vi "Bc&gfactor.vi"(4 "R square":cluster{dbl, dbl}[](graph)=[{-90000.0, 0.9936483367603044}, {-87906.97674418605, 0.9950094850030079}, {-85813.95348837209, 0.9957274737690295}, {-83720.93023255814, 0.9933108814011996}, {-81627.90697674418, 0.992357867872986}, {-79534.88372093023, 0.9862292416058566}, {-77441.86046511628, 0.99627541563675}, {-75348.83720930232, 0.9780001446047889}, {-73255.81395348837, 0.9762525196246166}, {-71162.79069767441, 0.9805623164953412}, {-69069.76744186046, 0.9733364259427615}, {-66976.7441860465, 0.9866906891307189}, {-64883.72093023256, 0.9887677477278096}, {-62790.6976744186, 0.9647771076841904}, {-60697.67441860465, 0.9547794787863182}, {-58604.651162790695, 0.9942809429807753}, {-56511.62790697674, 0.9851661179243407}, {-54418.60465116279, 0.9686064936549159}, {-52325.58139534883, 0.9659153710307546}, {-50232.55813953488, 0.9617268214492714}, {-48139.534883720924, 0.9756720636568874}, {-46046.51162790697, 0.9839504663053658}, {-43953.488372093016, 0.9970014960760687}, {-41860.46511627906, 0.9884092692332003}, {-39767.441860465115, 0.9866795475083417}, {-37674.41860465116, 0.9905062595043629}, {-35581.395348837206, 0.9798470326477143}, {-33488.37209302325, 0.9763040209572704}, {-31395.348837209298, 0.9974412233607519}, {-29302.325581395344, 0.9790950602168367}, {-27209.30232558139, 0.985787657243487}, {-25116.279069767435, 0.994663632255808}, {-23023.25581395348, 0.9948455965833045}, {-20930.232558139527, 0.9957582677028887}, {-18837.209302325573, 0.9958266077752963}, {-16744.18604651162, 0.9907170020986631}, {-14651.162790697665, 0.9943927190181459}, {-12558.13953488371, 0.9926116840879449}, {-10465.116279069756, 0.9936118308328861}, {-8372.093023255802, 0.993852544818158}, {-6279.069767441848, 0.991095330580116}, {-4186.046511627894, 0.9915888136201866}, {-2093.0232558139396, 0.9952686470079972}, {1.4551915228366852e-11, 0.9951187760658085}, {2093.0232558139687, 0.9938327422163827}, {4186.046511627923, 0.9949656993934944}, {6279.069767441877, 0.9912005637296157}, {8372.093023255831, 0.9916696176817267}, {10465.11627906977, 0.9922195047323839}, {12558.139534883725, 0.9929868887027957}, {14651.16279069768, 0.9900196190607464}, {16744.186046511633, 0.9944283927116259}, {18837.209302325587, 0.9940419981816503}, {20930.23255813954, 0.9927548489146202}, {23023.255813953496, 0.9936445754738522}, {25116.27906976745, 0.9980677514433665}, {27209.302325581404, 0.9960253172243516}, {29302.32558139536, 0.9927559692084316}, {31395.348837209312, 0.9773515443784792}, {33488.37209302327, 0.9897212577220764}, {35581.39534883722, 0.9924602641830366}, {37674.418604651175, 0.9791788400015979}, {39767.44186046513, 0.9788017425910343}, {41860.46511627908, 0.9808865900675626}, {43953.48837209304, 0.9789571284233267}, {46046.51162790699, 0.9671045339132186}, {48139.534883720946, 0.9672112912864314}, {50232.5581395349, 0.9665854302890936}, {52325.581395348854, 0.9620995151108727}, {54418.60465116281, 0.9860375825085537}, {56511.62790697676, 0.9877298129618225}, {58604.65116279072, 0.9625519591858813}, {60697.67441860467, 0.9721292461291907}, {62790.697674418625, 0.9759515933730254}, {64883.72093023258, 0.9762546173916274}, {66976.74418604653, 0.9914257931857835}, {69069.76744186049, 0.9589212650542382}, {71162.79069767444, 0.7584191634223125}, {73255.8139534884, 0.975789027366707}, {75348.83720930235, 0.9825220775303888}, {77441.8604651163, 0.9890951437370847}, {79534.88372093026, 0.9695146827415762}, {81627.90697674421, 0.9879709487631367}, {83720.93023255817, 0.9877215091218606}, {85813.95348837212, 0.9938806771671042}, {87906.97674418607, 0.9847409146593209}], 8 "Coupling factor error":dbl, 9 "Coupling factor (eV/V)":dbl=0.1, 10 "Which splitting?":i32, 11 "XY Graph 4":cluster{dbl[], dbl[]}[](graph)=[{[-0.02736853412017211, -0.02736853412017211, -0.027457159682098792, -0.02714680119515219, -0.027446691867251106, -0.02737107022650992, -0.027461949140044236, -0.027256401341539064, -0.026844150670273844, -0.027419393193521695, -0.027303914098034662, -0.02703602857347208, -0.026888259949045673, -0.026790317754302132, -0.026790317754302132, -0.026707850548493665, -0.026570137455754914, -0.026515227867687362, -0.026658413988083815, -0.02635338740252281, -0.026267451338723564, -0.026280953558885083, -0.026109172200008007, -0.025812412430651806, -0.02584267749186701, -0.02582141266526132, -0.025807417699267175, -0.025801332345852277, -0.025821043911205325, -0.025805086007194167, -0.025791278388417656, -0.025772190934840334, -0.02548288242077668, -0.025336678648638575, -0.02567859725920492, -0.0251601862977569, -0.025085545468475877, -0.025013386768161117, -0.024935335121923342, -0.02736853412017211, -0.027457159682098792, -0.027574435649012727, -0.027554636167478386, -0.027551280185925644, -0.02791992364189102, -0.027503183763744384, -0.027618288300652723, -0.027446691867251106, -0.0277547695215205, -0.02760603475092372, -0.027461949140044236, -0.027522335544211626, -0.027503918369851946, -0.027419393193521695, -0.027303914098034662, -0.028033474343692046, -0.02804592066528165, -0.028006221411939727, -0.028006221411939727, -0.028207245954529003, -0.028279854967391334, -0.028432698354546673, -0.028674911642963354, -0.028695367509489752, -0.028788991538842516, -0.028859733108892546, -0.028885909800132156, -0.02931385357599471, -0.02883940989296912, -0.029107906174069182, -0.02914731021476181, -0.02920151841150575, -0.02863587278290227, -0.0295034906955593, -0.02997153941497236, -0.029743359934365898, -0.029820070650600022, -0.02951890711445811, -0.029555073471882756, -0.03004045441204873, -0.030156155658522733, -0.03027418428153998, -0.03011762696127086, -0.02736853412017211, -0.02757948642923058, -0.027610051126103378, -0.02764371579608451, -0.02756195552606243, -0.027634391513683045, -0.0275993752474062, -0.027127858278431297, -0.027440893163395392, -0.02744279598938577, -0.0275929298338454, -0.027591913990705083, -0.027565176585148243, -0.027533400296601417, -0.027330808874349643, -0.026744397861130295, -0.026982223848265225, -0.0269200804791046, -0.026856856233696994, -0.026700905436478503, -0.026700905436478503, -0.026665888611385614, -0.026544473254661284, -0.026445905848945565, -0.026338442772813758, -0.026263987266378474, -0.026551732521948368, -0.025944373776851146, -0.026112993018050888, -0.025889198816972006, -0.02586884204773503, -0.02588741873327973, -0.02585416095870263, -0.025896027615352635, -0.02588651620829451, -0.025899204618664493, -0.02586615626570455, -0.025770624667800432, -0.025703440860855863, -0.025747957866592296, -0.02535208231276207, -0.0252641528372817, -0.02521204130779185, -0.025156133749437332, -0.028319357512760632, -0.028373870368935062, -0.02800141524302324, -0.02756195552606243, -0.027634391513683045, -0.0275993752474062, -0.027689782895953863, -0.027826807607735864, -0.027950048307487676, -0.0275929298338454, -0.027591913990705083, -0.027565176585148243, -0.027533400296601417, -0.028298889889664804, -0.028307392754636704, -0.0283834573520277, -0.028475963804310153, -0.028508912222203024, -0.028508912222203024, -0.028646314658785015, -0.028200351086857745, -0.0287555540748013, -0.02873971887513881, -0.028779787878370027, -0.029072053575197022, -0.02895116220904841, -0.029287108790671378, -0.029178204968174144, -0.029322294689052453, -0.029417108027244444, -0.029433069816662265, -0.02962878437629653, -0.029718349543882774, -0.029788089545410783, -0.02987921181622441, -0.029600956616660113, -0.02905050167349195, -0.02917031235640807, -0.03011604320884724, -0.030126554480480978, -0.030182798802889002, -0.030209271213091124], [0.0, 1.4551915228366852e-11, 2093.0232558139687, 14651.16279069768, 16744.186046511633, 18837.209302325587, 23023.255813953496, 25116.27906976745, 27209.302325581404, 29302.32558139536, 31395.348837209312, 33488.37209302327, 35581.39534883722, 37674.418604651175, 37674.418604651175, 39767.44186046513, 41860.46511627908, 43953.48837209304, 46046.51162790699, 48139.534883720946, 50232.5581395349, 52325.581395348854, 54418.60465116281, 56511.62790697676, 58604.65116279072, 60697.67441860467, 62790.697674418625, 64883.72093023258, 66976.74418604653, 69069.76744186049, 71162.79069767444, 73255.8139534884, 75348.83720930235, 77441.8604651163, 79534.88372093026, 81627.90697674421, 83720.93023255817, 85813.95348837212, 87906.97674418607, 1.4551915228366852e-11, 2093.0232558139687, 4186.046511627923, 6279.069767441877, 8372.093023255831, 10465.11627906977, 12558.139534883725, 14651.16279069768, 16744.186046511633, 18837.209302325587, 20930.23255813954, 23023.255813953496, 25116.27906976745, 27209.302325581404, 29302.32558139536, 31395.348837209312, 33488.37209302327, 35581.39534883722, 37674.418604651175, 37674.418604651175, 39767.44186046513, 41860.46511627908, 43953.48837209304, 46046.51162790699, 48139.534883720946, 50232.5581395349, 52325.581395348854, 54418.60465116281, 56511.62790697676, 58604.65116279072, 60697.67441860467, 62790.697674418625, 64883.72093023258, 66976.74418604653, 69069.76744186049, 71162.79069767444, 73255.8139534884, 75348.83720930235, 77441.8604651163, 79534.88372093026, 81627.90697674421, 83720.93023255817, 85813.95348837212, 87906.97674418607, 0.0, -2093.0232558139396, -4186.046511627894, -6279.069767441848, -10465.116279069756, -12558.13953488371, -14651.162790697665, -16744.18604651162, -18837.209302325573, -20930.232558139527, -23023.25581395348, -25116.279069767435, -27209.30232558139, -29302.325581395344, -31395.348837209298, -33488.37209302325, -35581.395348837206, -37674.41860465116, -39767.441860465115, -41860.46511627906, -41860.46511627906, -43953.488372093016, -46046.51162790697, -48139.534883720924, -50232.55813953488, -52325.58139534883, -54418.60465116279, -56511.62790697674, -58604.651162790695, -60697.67441860465, -62790.6976744186, -64883.72093023256, -66976.7441860465, -69069.76744186046, -71162.79069767441, -73255.81395348837, -75348.83720930232, -77441.86046511628, -79534.88372093023, -81627.90697674418, -83720.93023255814, -85813.95348837209, -87906.97674418605, -90000.0, -4186.046511627894, -6279.069767441848, -8372.093023255802, -10465.116279069756, -12558.13953488371, -14651.162790697665, -16744.18604651162, -18837.209302325573, -20930.232558139527, -23023.25581395348, -25116.279069767435, -27209.30232558139, -29302.325581395344, -31395.348837209298, -35581.395348837206, -37674.41860465116, -39767.441860465115, -41860.46511627906, -41860.46511627906, -43953.488372093016, -46046.51162790697, -48139.534883720924, -50232.55813953488, -52325.58139534883, -54418.60465116279, -56511.62790697674, -58604.651162790695, -60697.67441860465, -62790.6976744186, -64883.72093023256, -66976.7441860465, -69069.76744186046, -71162.79069767441, -73255.81395348837, -75348.83720930232, -77441.86046511628, -79534.88372093023, -81627.90697674418, -83720.93023255814, -85813.95348837209, -87906.97674418605, -90000.0]}]) -> (0 "g factor error":cluster{"g+ error":dbl, "g- error":dbl}={"g+ error"=0.0638565699892568, "g- error"=0.06800901914377956}, 1 "Bc error":T1={"Bc+ error (Oe)"=2088.9643668800263, "Bc- error (Oe)"=2622.097899688439}, 2 "g factor":cluster{"g+":dbl, "g-":dbl}={"g+"=1.3399908059362309, "g-"=1.1298275555458581}, 3 "Bc":cluster{"Bc+":dbl, "Bc-":dbl}={"Bc+"=20293.555386834036, "Bc-"=-14870.573041686936})   [LabVIEW 2013]
uses:
  <vilib>/Analysis/baseanly.llb/Mean (DBL).vi
  <vilib>/Analysis/NI_AALPro.lvlib
  <vilib>/Analysis/NI_AALBase.lvlib
panel:
  in  "R-square threshold":dbl(slide)=0.95 scale=0.95..1.0
  out "Vsg":dbl=-0.027570634803083107 format="%.3f"
  in  "Slide 2":cluster{dbl, dbl}(slide)={1.0, 0.0} scale=0.0..1.0
  in  "Slide":cluster{dbl, dbl}(slide)={0.9083969465648855, 0.13740458015267176} scale=0.0..1.0
  out "XY Graph 6":cluster{dbl[], dbl[]}[](graph)=[{[0.0034223544898157737, 0.003347060812636086, 0.003830331948859681, 0.00401305555051986, 0.0038888849267462895, 0.0038318333355882653, 0.003732756760943895, 0.003578908857959636, 0.0035296892939647127, 0.003453452641317422, 0.003289006151202138, 0.00317411577262049, 0.003006788432197264, 0.0025203210532486545, 0.0025158006119915532, 0.002401276102325052, 0.0023096482258557344, 0.001655877832196461, 0.001980426047399401, 0.001619107570613159, 0.0014633768729231007, 0.0013251689063714794, 0.0009680810153151614, 0.0005072523181019056, 0.00038591444434047176], [-81627.90697674418, -79534.88372093023, -77441.86046511628, -75348.83720930232, -73255.81395348837, -71162.79069767441, -69069.76744186046, -66976.7441860465, -64883.72093023256, -62790.6976744186, -60697.67441860465, -58604.651162790695, -56511.62790697674, -54418.60465116279, -52325.58139534883, -50232.55813953488, -48139.534883720924, -46046.51162790697, -43953.488372093016, -39767.441860465115, -37674.41860465116, -35581.395348837206, -31395.348837209298, -20930.232558139527, -18837.209302325573]}, {[0.0009974457702199672, 0.001157660716235978, 0.0014993954060353379, 0.0017097175116364202, 0.0019174704868593108, 0.0020164976548795385, 0.0023419801069669427, 0.002521540200118952, 0.002578779550007463, 0.0027767376001241496, 0.0035014411453429053, 0.0029967324011021083, 0.003286493508807862, 0.003339892515494637, 0.0034001860656534717, 0.0028148288716969457, 0.0036984046883651346, 0.003971168999525564, 0.004337188229823343, 0.004182228465819535, 0.0038764762126778374, 0.00488026811429183, 0.005070610190046856, 0.005260797513378865, 0.005182291839347517], [33488.37209302327, 35581.39534883722, 39767.44186046513, 41860.46511627908, 43953.48837209304, 46046.51162790699, 48139.534883720946, 50232.5581395349, 52325.581395348854, 54418.60465116281, 56511.62790697676, 58604.65116279072, 60697.67441860467, 62790.697674418625, 64883.72093023258, 66976.74418604653, 69069.76744186049, 73255.8139534884, 75348.83720930235, 77441.8604651163, 79534.88372093026, 81627.90697674421, 83720.93023255817, 85813.95348837212, 87906.97674418607]}]
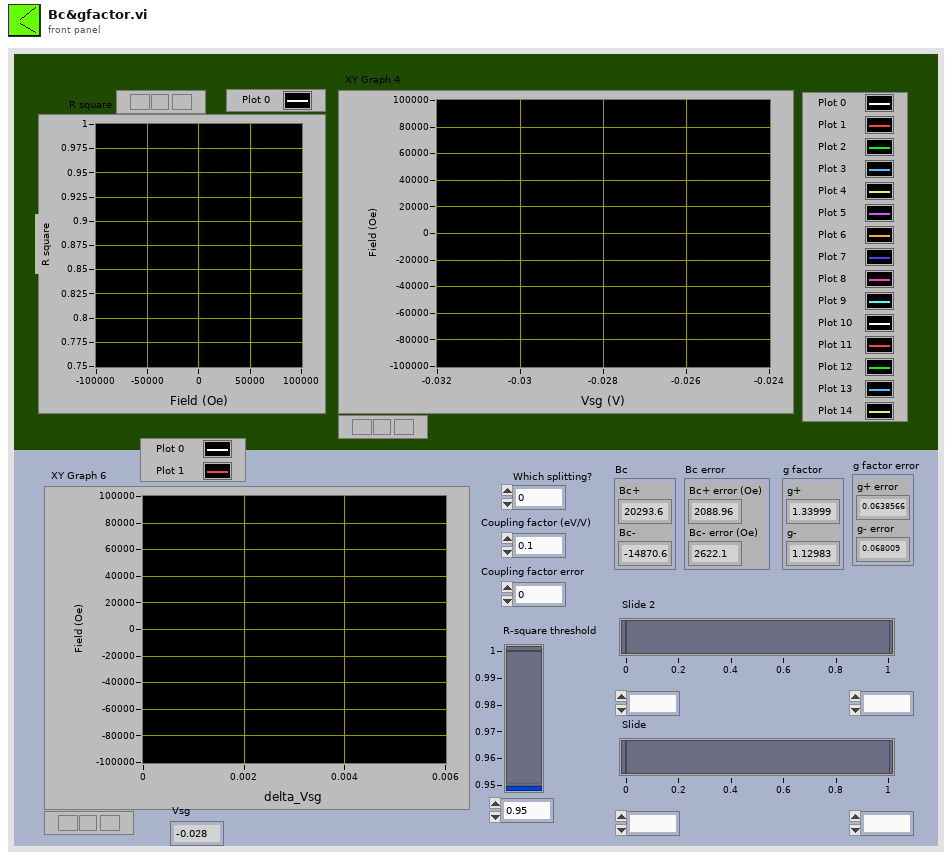
[diagram p1: front panel]
types:
  T1 = cluster{"Bc+ error (Oe)":dbl, "Bc- error (Oe)":dbl}
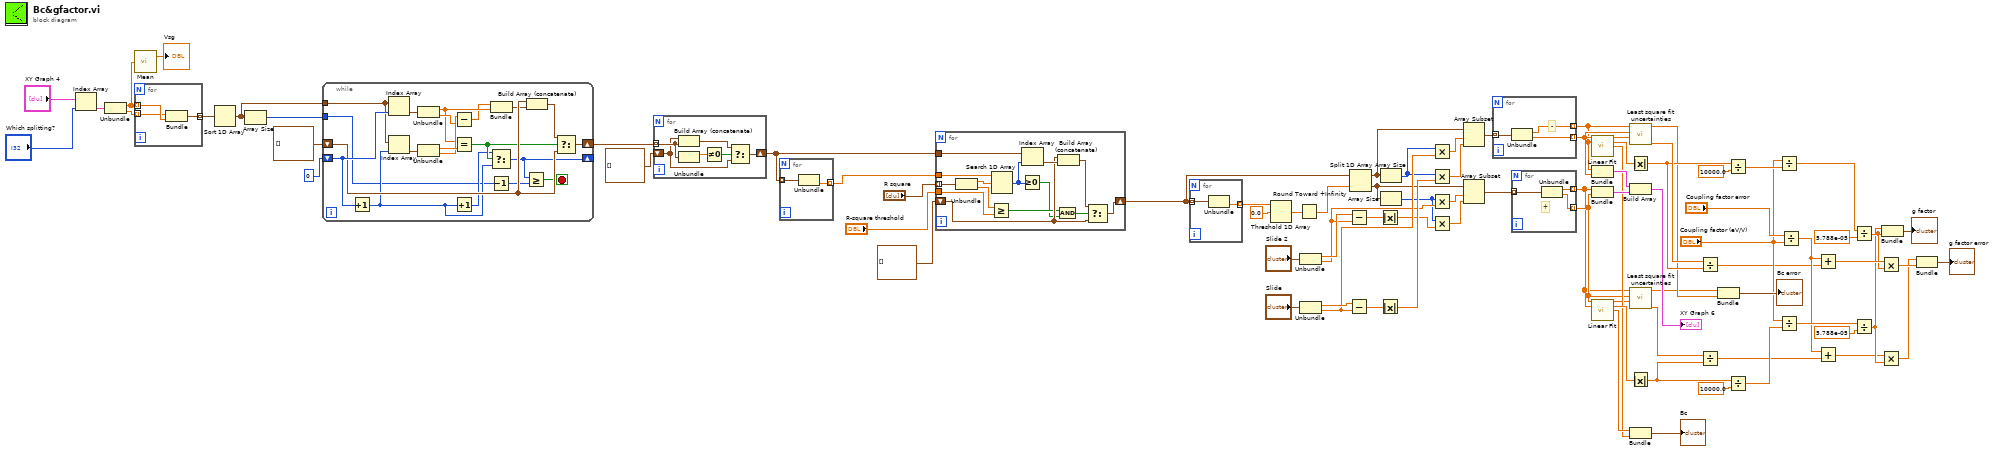
[diagram p0: block diagram]
diagram:
  n1 = Index Array(array="XY Graph 4", index="Which splitting?") -> (element=w83:cluster{dbl[], dbl[]})
  n2 = Unbundle(w83) -> (w36:dbl[], w82:dbl[])
  n3 = call-poly <vilib>:"Mean.vi"("X"=w36) -> ("mean"=→"Vsg":dbl)  [unwired: 1 out]
  n4 = for {
    tunnel: w36 -> [w88] mode=indexing
    tunnel: w82 -> [w87] mode=indexing
    tunnel: [w86] -> w81 mode=indexing
    n5 = Bundle(w87, w88) -> (w86:cluster{dbl, dbl})  [unwired: 1 in]
  }
  n6 = Sort 1D Array(array=w81) -> (sorted array=w77:cluster{dbl, dbl}[])
  n7 = Array Size(array=w77) -> (size(s)=w78:i32)
  n8 = while {
    tunnel: w77 -> [w107]
    shift-right: [w95] -> _
    shift-left: 0 -> [w108]
    shift-right: [w100] -> w75
    shift-left: cluster{dbl, dbl}[] [] -> [w99]
    tunnel: w78 -> [w94]
    stop <- w92 stop-if-true
    n9 = Increment(x=w108) -> (x+1=w96:i32)
    n10 = Index Array(array=w107, index=w108) -> (element=w106:cluster{dbl, dbl})
    n11 = Index Array(array=w107, index=w96) -> (element=w105:cluster{dbl, dbl})
    n12 = Unbundle(w106) -> (w91:dbl, w102:dbl)
    n13 = Unbundle(w105) -> (w104:dbl, w103:dbl)
    n14 = Subtract(x=w103, y=w102) -> (x-y=w90:dbl)
    n15 = Equal?(x=w91, y=w104) -> (x = y?=w98:bool)
    n16 = Increment(x=w96) -> (x+1=w97:i32)
    n17 = Decrement(x=w94) -> (x-1=w93:i32)
    n18 = Bundle(w90, w91) -> (w89:cluster{dbl, dbl})  [unwired: 1 in]
    n19 = Select(t=w97, s=w98, f=w96) -> (s? t:f=w95:i32)
    n20 = Greater Or Equal?(x=w95, y=w93) -> (x >= y?=w92:bool)
    n21 = Build Array (concatenate)(w99, w89) -> (w101:cluster{dbl, dbl}[])
    n22 = Select(t=w101, s=w98, f=w99) -> (s? t:f=w100:cluster{dbl, dbl}[])
  }
  n23 = for {
    tunnel: w75 -> [w113] mode=indexing
    shift-right: [w111] -> w1
    shift-left: cluster{dbl, dbl}[] [] -> [w110]
    n24 = Build Array (concatenate)(w110, w113) -> (w112:cluster{dbl, dbl}[])
    n25 = Unbundle(w113) -> (w109:dbl)  [unwired: 1 out]
    n26 = Not Equal To 0?(x=w109) -> (x != 0?=w114:bool)
    n27 = Select(t=w112, s=w114, f=w110) -> (s? t:f=w111:cluster{dbl, dbl}[])
  }
  n28 = for {
    tunnel: w1 -> [w116] mode=indexing
    tunnel: [w115] -> w4 mode=indexing
    n29 = Unbundle(w116) -> (w115:dbl)  [unwired: 1 out]
  }
  n30 = for {
    tunnel: "R square" -> [w130] mode=indexing
    tunnel: "R-square threshold" -> [w128]
    tunnel: w4 -> [w126]
    shift-right: [w122] -> w2
    shift-left: cluster{dbl, dbl}[] [] -> [w121]
    tunnel: w1 -> [w125]
    n31 = Unbundle(w130) -> (w127:dbl, w129:dbl)
    n32 = Greater Or Equal?(x=w129, y=w128) -> (x >= y?=w119:bool)
    n33 = Search 1D Array(1D array=w126, element=w127) -> (index of element=w120:i32)  [unwired: 1 in]
    n34 = Greater Or Equal To 0?(x=w120) -> (x >= 0?=w118:bool)
    n35 = Index Array(array=w125, index=w120) -> (element=w124:cluster{dbl, dbl})
    n36 = And(x=w119, y=w118) -> (x .and. y?=w117:bool)
    n37 = Build Array (concatenate)(w121, w124) -> (w123:cluster{dbl, dbl}[])
    n38 = Select(t=w123, s=w117, f=w121) -> (s? t:f=w122:cluster{dbl, dbl}[])
  }
  n39 = for {
    tunnel: w2 -> [w132] mode=indexing
    tunnel: [w131] -> w74 mode=indexing
    n40 = Unbundle(w132) -> (w131:dbl)  [unwired: 1 out]
  }
  n41 = Threshold 1D Array(2:0.0 ("threshold y"), 3:w74) -> (0:w72:dbl)  [unwired: 1 in]
  n42 = Round Toward +Infinity(x=w72) -> (ceil(x): smallest int >= x=w71:dbl)
  n43 = Unbundle("Slide 2") -> (w57:dbl, w55:dbl)
  n44 = Unbundle("Slide") -> (w67:dbl, w65:dbl)
  n45 = Subtract(x=w57, y=w55) -> (x-y=w56:dbl)
  n46 = Subtract(x=w67, y=w65) -> (x-y=w66:dbl)
  n47 = Split 1D Array(array=w2, index=w71) -> (first subarray=w59:cluster{dbl, dbl}[], second subarray=w49:cluster{dbl, dbl}[])
  n48 = Absolute Value(x=w56) -> (abs(x)=w53:dbl)
  n49 = Absolute Value(x=w66) -> (abs(x)=w63:dbl)
  n50 = Array Size(array=w59) -> (size(s)=w64:i32)
  n51 = Array Size(array=w49) -> (size(s)=w54:i32)
  n52 = Multiply(x=w64, y=w65) -> (x*y=w61:dbl)
  n53 = Multiply(x=w64, y=w63) -> (x*y=w62:dbl)
  n54 = Multiply(x=w54, y=w55) -> (x*y=w51:dbl)
  n55 = Multiply(x=w54, y=w53) -> (x*y=w52:dbl)
  n56 = Array Subset(array=w59, index=w61, length=w62) -> (w58:cluster{dbl, dbl}[])
  n57 = Array Subset(array=w49, index=w51, length=w52) -> (w48:cluster{dbl, dbl}[])
  n58 = for {
    tunnel: w58 -> [w135] mode=indexing
    tunnel: [w134] -> w33 mode=indexing
    tunnel: [w133] -> w34 mode=indexing
    # "-"
    n59 = Unbundle(w135) -> (w134:dbl, w133:dbl)
  }
  n60 = for {
    tunnel: w48 -> [w138] mode=indexing
    tunnel: [w137] -> w30 mode=indexing
    tunnel: [w136] -> w31 mode=indexing
    # "+"
    n61 = Unbundle(w138) -> (w137:dbl, w136:dbl)
  }
  n62 = call <vilib>:"Linear Fit.vi"("Y"=w34, "X"=w33) -> ("Best Linear Fit"=w32:dbl[], "slope"=w47:dbl, "intercept"=w39:dbl)  [unwired: 9 in, 2 out]
  n63 = Bundle(w33, w34) -> (w70:cluster{dbl[], dbl[]})  [unwired: 1 in]
  n64 = Bundle(w30, w31) -> (w69:cluster{dbl[], dbl[]})  [unwired: 1 in]
  n65 = call <vilib>:"Linear Fit.vi"("Y"=w31, "X"=w30) -> ("Best Linear Fit"=w29:dbl[], "slope"=w41:dbl, "intercept"=w40:dbl)  [unwired: 9 in, 2 out]
  n66 = call <userlib>:"Least square fit uncertainties.vi"("Best Linear Fit"=w32, "Y"=w34, "X"=w33) -> ("sigma_B (Oe/V)"=w19:dbl, "sigma_A (Oe)"=w16:dbl)  [unwired: 7 in]
  n67 = Absolute Value(x=w47) -> (abs(x)=w18:dbl)
  n68 = Build Array(w70, w69) -> (→"XY Graph 6":cluster{dbl[], dbl[]}[])
  n69 = call <userlib>:"Least square fit uncertainties.vi"("Best Linear Fit"=w29, "Y"=w31, "X"=w30) -> ("sigma_B (Oe/V)"=w26:dbl, "sigma_A (Oe)"=w15:dbl)  [unwired: 7 in]
  n70 = Absolute Value(x=w41) -> (abs(x)=w25:dbl)
  n71 = Bundle("intercept"=w40, "intercept"=w39) -> (→"Bc":cluster{"intercept":dbl, "intercept":dbl})  [unwired: 1 in]
  n72 = Divide(x=w19, y=w18) -> (x/y=w17:dbl)
  n73 = Divide(x=w26, y=w25) -> (x/y=w21:dbl)
  n74 = Bundle("sigma_A (Oe)"=w15, "sigma_A (Oe)"=w16) -> (→"Bc error":cluster{"sigma_A (Oe)":dbl, "sigma_A (Oe)":dbl})  [unwired: 1 in]
  n75 = Divide(x=w18, y=10000.0) -> (x/y=w45:dbl)
  n76 = Divide(x=w25, y=10000.0) -> (x/y=w28:dbl)
  n77 = Divide(x="Coupling factor (eV/V)", y=w45) -> (x/y=w13:dbl)
  n78 = Divide(x="Coupling factor (eV/V)", y=w28) -> (x/y=w42:dbl)
  n79 = Divide(x="Coupling factor error", y="Coupling factor (eV/V)") -> (x/y=w20:dbl)
  n80 = Add(x=w20, y=w17) -> (x+y=w14:dbl)
  n81 = Add(x=w20, y=w21) -> (x+y=w9:dbl)
  n82 = Divide(x=w13, y=5.788e-05) -> (x/y=w11:dbl)
  n83 = Divide(x=w42, y=5.788e-05) -> (x/y=w10:dbl)
  n84 = Multiply(x=w14, y=w11) -> (x*y=w12:dbl)
  n85 = Multiply(x=w9, y=w10) -> (x*y=w8:dbl)
  n86 = Bundle(w10, w11) -> (→"g factor":cluster{dbl, dbl})  [unwired: 1 in]
  n87 = Bundle(w8, w12) -> (→"g factor error":cluster{dbl, dbl})  [unwired: 1 in]
